vi "Register gRPC Methods.vi"(8 "error in (no error)":errorcluster, 11 "Template Server in":refnum<class "MeasurementService.lvclass">) -> (0 "error out":errorcluster, 3 "Template Server out":refnum<class "MeasurementService.lvclass">)   [LabVIEW 2021, in "Measurement_server.lvlib" / "MeasurementService.lvclass"]
uses:
  MeasurementService.lvclass
  typeDefs/Server Internal UEs.ctl
  typeDefs/Server Internal Message.ctl
  typeDefs/Server gRPC UEs.ctl
  <vilib>/gRPC/LabVIEW gRPC Library/Server API/typeDefs/gRPCId Cluster.ctl
  <vilib>/gRPC/LabVIEW gRPC Library/Shared/grpcId.ctl
  MeasurementService.lvclass/MeasurementService.ctl
  <vilib>/gRPC/LabVIEW gRPC Library/grpc-lvsupport-release.lvlib
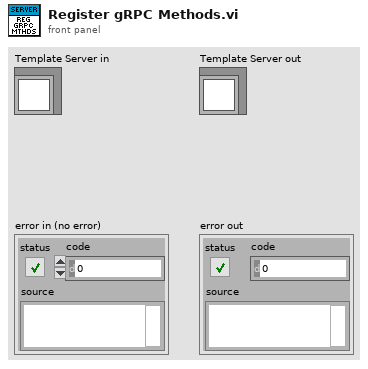
[diagram p1: front panel]
types:
  T1 = typedef "Measurement_server.lvlib/MeasurementService.lvclass/Server gRPC UEs.ctl" = cluster{"MeasurementService GetStatus gRPC UE":refnum<user-event>, "MeasurementService AcquireSensorData gRPC UE":refnum<user-event>, "MeasurementService ProcessData gRPC UE":refnum<user-event>, "MeasurementService StreamSensorData gRPC UE":refnum<user-event>}
  T2 = typedef "Measurement_server.lvlib/MeasurementService.lvclass/Server Internal UEs.ctl" = cluster{"MeasurementService GetStatus Internal UE":refnum<user-event>, "MeasurementService AcquireSensorData Internal UE":refnum<user-event>, "MeasurementService ProcessData Internal UE":refnum<user-event>, "MeasurementService StreamSensorData Internal UE":refnum<user-event>}
  T3 = typedef "grpc-lvsupport-release.lvlib/grpcId.ctl" = u64
  T4 = typedef "Measurement_server.lvlib/MeasurementService.lvclass/Server Internal Message UE.ctl" = refnum<user-event>
  T5 = typedef "grpc-lvsupport-release.lvlib/gRPCId Cluster UE.ctl" = refnum<user-event>
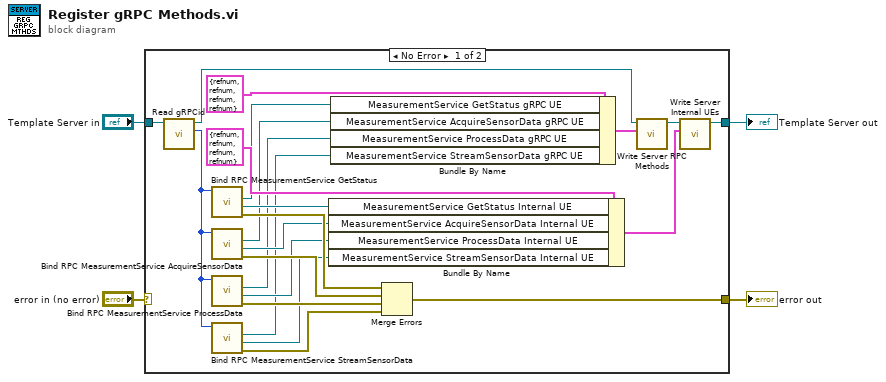
[diagram p0: block diagram]
diagram:
  n1 = case shown="No Error" "error in (no error)" {
    selector: "error in (no error)" -> [_ w27]
    tunnel: "Template Server in" -> [w18 w28]
    tunnel: [w26 w27] -> w3
    tunnel: [w25 w28] -> w2
    frame No Error {
      n2 = call-dynamic "Read gRPCid.vi"("iService in"=w18) -> ("gRPCid"=w17:T3, "iService out"=w19:refnum<class "MeasurementService.lvclass">)  [unwired: 8 in, 1 out]
      n3 = call "Bind RPC MeasurementService GetStatus.vi"("gRPCid server in"=w17) -> ("error out"=w16:errorcluster, "MeasurementService GetStatus Internal UE"=w14:T4, "MeasurementService GetStatus gRPC UE"=w15:T5)  [unwired: 7 in, 1 out]
      n4 = call "Bind RPC MeasurementService AcquireSensorData.vi"("gRPCid server in"=w17) -> ("error out"=w13:errorcluster, "MeasurementService AcquireSensorData Internal UE"=w11:T4, "MeasurementService AcquireSensorData gRPC UE"=w12:T5)  [unwired: 7 in, 1 out]
      n5 = call "Bind RPC MeasurementService ProcessData.vi"("gRPCid server in"=w17) -> ("error out"=w10:errorcluster, "MeasurementService ProcessData Internal UE"=w8:T4, "MeasurementService ProcessData gRPC UE"=w9:T5)  [unwired: 7 in, 1 out]
      n6 = call "Bind RPC MeasurementService StreamSensorData.vi"("gRPCid server in"=w17) -> ("error out"=w7:errorcluster, "MeasurementService StreamSensorData Internal UE"=w5:T4, "MeasurementService StreamSensorData gRPC UE"=w6:T5)  [unwired: 7 in, 1 out]
      n7 = Bundle By Name ("Bundle Internal UEs")(cluster=T2 {"MeasurementService GetStatus Internal UE"=refnum, "MeasurementService AcquireSensorData Internal UE"=refnum, "MeasurementService ProcessData Internal UE"=refnum, "MeasurementService StreamSensorData Internal UE"=refnum} ("Server Internal UEs"), "MeasurementService GetStatus Internal UE"=w14, "MeasurementService AcquireSensorData Internal UE"=w11, "MeasurementService ProcessData Internal UE"=w8, "MeasurementService StreamSensorData Internal UE"=w5) -> (w24:T2)
      n8 = Bundle By Name ("Bundle gRPC UEs")(cluster=T1 {"MeasurementService GetStatus gRPC UE"=refnum, "MeasurementService AcquireSensorData gRPC UE"=refnum, "MeasurementService ProcessData gRPC UE"=refnum, "MeasurementService StreamSensorData gRPC UE"=refnum} ("gRPC Server Method Events"), "MeasurementService GetStatus gRPC UE"=w15, "MeasurementService AcquireSensorData gRPC UE"=w12, "MeasurementService ProcessData gRPC UE"=w9, "MeasurementService StreamSensorData gRPC UE"=w6) -> (w21:T1)
      n9 = Merge Errors(w16, w13, w10, w7) -> (w26:errorcluster)
      n10 = call "Write Server RPC Methods.vi"("Server RPC Methods"=w21, "SignalGeneratorService in"=w19) -> ("SignalGeneratorService out"=w22:refnum<class "MeasurementService.lvclass">)  [unwired: 8 in, 1 out]
      n11 = call "Write Server Internal UEs.vi"("Server Internal UEs"=w24, "SignalGeneratorService in"=w22) -> ("SignalGeneratorService out"=w25:refnum<class "MeasurementService.lvclass">)  [unwired: 8 in, 1 out]
    }
    frame Error {
    }
  }
  "error out" <- w3
  "Template Server out" <- w2
